vi "Validate Incoming Packet.vi"(8 "error in (no error)":errorcluster, 10 "ControlPacket":refnum<class "ControlPacket.lvclass">, 11 "Session.Server in":refnum<class "Session.Server.lvclass">) -> (0 "error out":errorcluster, 2 "ControlPacket out":refnum<class "ControlPacket.lvclass">, 3 "Session.Server out":refnum<class "Session.Server.lvclass">)   [LabVIEW 2013, in "MQTT Server.lvlib" / "Session.Server.lvclass"]
uses:
  Session.Server.lvclass
  <vilib>/LabVIEW Open Source Project/MQTT Control Packets/Control Packets/ControlPacket/ControlPacket.lvclass
  Session.Server.lvclass/Session.Server.ctl
  <vilib>/LabVIEW Open Source Project/MQTT Control Packets/Control Packets/CONNECT/CONNECT.lvclass
  MQTT_Base/Session/Session.lvclass/Session.ctl
  MQTT_Base/Session/Session.lvclass
  <vilib>/LabVIEW Open Source Project/MQTT Control Packets/Control Packets/SUBSCRIBE/SUBSCRIBE.lvclass
  StoredSessions/StoredSessions.lvclass
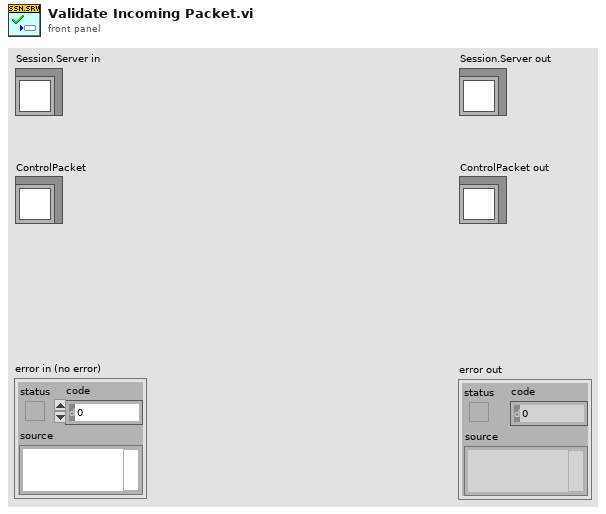
[diagram p1: front panel]
types:
  T1 = typedef "MQTT_Control_Packets.lvlib/ControlPacket.lvclass/Control Packet Type -- enum.ctl" = enum16{"Reserved", "CONNECT", "CONNACK", "PUBLISH", "PUBACK", "PUBREC", "PUBREL", "PUBCOMP", "SUBSCRIBE", "SUBACK", "UNSUBSCRIBE", "UNSUBACK", "PINGREQ", "PINGRESP", "DISCONNECT", "AUTH"}
  T2 = typedef "MQTT_Control_Packets.lvlib/CONNECT.lvclass/ConnectFlags -- cluster.ctl" = cluster{"Reserved":bool, "Clean Session":bool, "Will Flag":bool, "Will QoS 1":bool, "Will QoS 2":bool, "Will Retain":bool, "Password Flag":bool, "User Name Flag":bool}
  T3 = typedef "MQTT_Control_Packets.lvlib/SUBSCRIBE.lvclass/Topic Subscription -- cluster.ctl" = cluster{"Topic Filter":string, "QoS":T4}
  T4 = typedef "MQTT_Control_Packets.lvlib/ControlPacket.lvclass/QualityOfService -- enum.ctl" = enum16{"0 (At Most Once)", "1 (At Least Once)", "2 (Exactly Once)"}
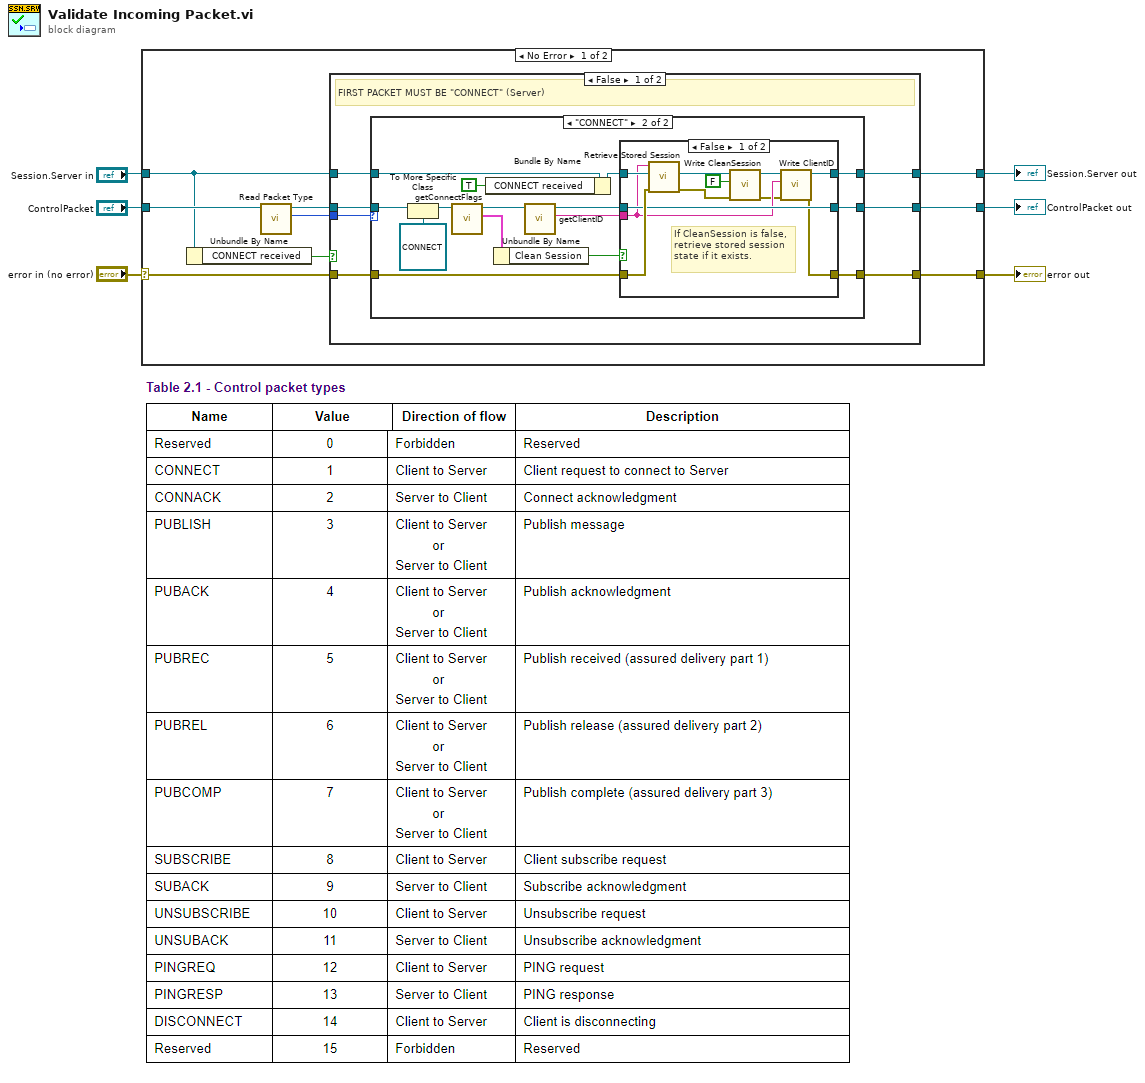
[diagram p0: block diagram]
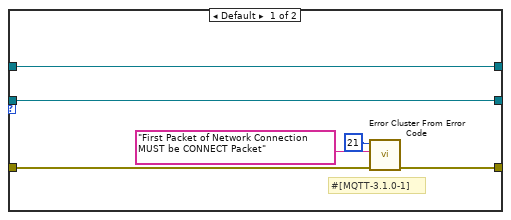
[diagram p2: hidden frame]
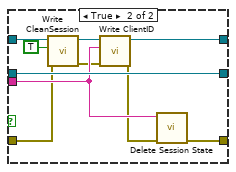
[diagram p3: hidden frame]
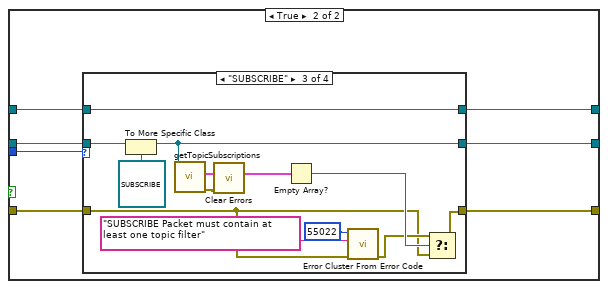
[diagram p4: hidden frame]
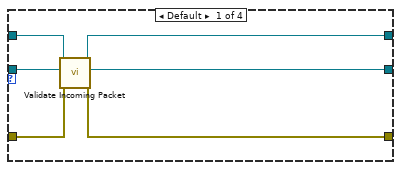
[diagram p5: hidden frame]
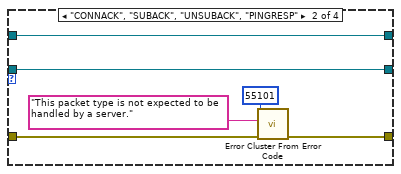
[diagram p6: hidden frame]
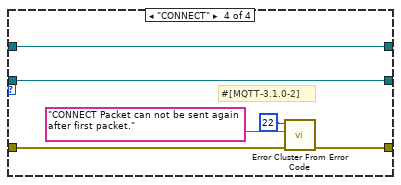
[diagram p7: hidden frame]
diagram:
  n1 = case shown="No Error" "error in (no error)" {
    selector: "error in (no error)" -> [w12 w104]
    tunnel: [w11 w104] -> w1
    tunnel: [w13 w103] -> w3
    tunnel: "Session.Server in" -> [w10 w103]
    tunnel: "ControlPacket" -> [w14 w102]
    tunnel: [w15 w102] -> w2
    frame No Error {
      n2 = Unbundle By Name(w10) -> ("CONNECT received"=w9:bool)
      n3 = call <vilib>:"Read Packet Type.vi"("ControlPacket in"=w14) -> ("Control Packet Type"=w7:T1, "ControlPacket out"=w8:refnum<class "ControlPacket.lvclass">)  [unwired: 9 in]
      n4 = case shown="False" w9 {
        tunnel: w8 -> [w16 w70]
        tunnel: [w17 w69] -> w15
        tunnel: w10 -> [w19 w66]
        tunnel: w7 -> [w20 w71]
        tunnel: [w18 w65] -> w13
        tunnel: w12 -> [w22 w68]
        tunnel: [w21 w67] -> w11
        frame False {
          # "FIRST PACKET MUST BE \"CONNECT\" (Server)"
          n5 = case shown="\"CONNECT\"" w20 {
            tunnel: w22 -> [w27 w32]
            tunnel: [w28 w33] -> w21
            tunnel: w19 -> [w26 w43]
            tunnel: [w26 w36] -> w18
            tunnel: [w25 w34] -> w17
            tunnel: w16 -> [w25 w40]
            frame Default {
              # "#[MQTT-3.1.0-1]"
              n6 = call <vilib>:"Error Cluster From Error Code.vi"("error in (no error)"=w27, "error message (\"\")"="First Packet of Network Connection MUST be CONNECT Packet", "error code (0)"=21) -> ("error out"=w28:errorcluster)  [unwired: 6 in]
            }
            frame "CONNECT" {
              n7 = To More Specific Class(target class=refnum<class "CONNECT.lvclass"> refnum ("CONNECT.lvclass"), reference=w40) -> (specific class reference=w39:refnum<class "CONNECT.lvclass">)  [unwired: 1 in, 1 out]
              n8 = call <vilib>:"getConnectFlags.vi"("CONNECT in"=w39) -> ("Connect Flags"=w38:T2, "CONNECT out"=w31:refnum<class "CONNECT.lvclass">)  [unwired: 9 in]
              n9 = Bundle By Name(cluster=w43, "CONNECT received"=TRUE) -> (w35:refnum<class "Session.Server.lvclass">)
              n10 = Unbundle By Name(w38) -> ("Clean Session"=w37:bool)
              n11 = call <vilib>:"getClientID.vi"("CONNECT in"=w31) -> ("Client ID"=w29:string, "CONNECT out"=w30:refnum<class "CONNECT.lvclass">)  [unwired: 9 in]
              n12 = case shown="False" w37 {
                tunnel: w30 -> [w50 w64]
                tunnel: [w47 w58] -> w36
                tunnel: w35 -> [w54 w62]
                tunnel: [w50 w64] -> w34
                tunnel: [w44 w63] -> w33
                tunnel: w32 -> [w52 w56]
                tunnel: w29 -> [w46 w60]
                frame False {
                  # "If CleanSession is false,\nretrieve stored session\nstate if it exists."
                  n13 = call "Retrieve Stored Session.vi"("error in (no error)"=w52, "Session in"=w54, "Client ID"=w46) -> ("error out"=w51:errorcluster, "Retrieved Session"=w53:refnum<class "Session.Server.lvclass">)  [unwired: 6 in, 1 out]
                  n14 = call "Write CleanSession.vi"("error in (no error)"=w51, "CleanSession"=FALSE, "Session in"=w53) -> ("error out"=w45:errorcluster, "Session out"=w48:refnum<class "Session.Server.lvclass">)  [unwired: 7 in]
                  n15 = call "Write ClientID.vi"("error in (no error)"=w45, "Client ID"=w46, "Session in"=w48) -> ("error out"=w44:errorcluster, "Session out"=w47:refnum<class "Session.Server.lvclass">)  [unwired: 7 in]
                }
                frame True {
                  n16 = call "Write CleanSession.vi"("error in (no error)"=w56, "CleanSession"=TRUE, "Session in"=w62) -> ("error out"=w57:errorcluster, "Session out"=w59:refnum<class "Session.Server.lvclass">)  [unwired: 7 in]
                  n17 = call "Write ClientID.vi"("error in (no error)"=w57, "Client ID"=w60, "Session in"=w59) -> ("error out"=w55:errorcluster, "Session out"=w58:refnum<class "Session.Server.lvclass">)  [unwired: 7 in]
                  n18 = call "Delete Session State.vi"("error in (no error)"=w55, "Client ID"=w60) -> ("error out"=w63:errorcluster)  [unwired: 9 in]
                }
              }
            }
          }
        }
        frame True {
          n19 = case shown="\"SUBSCRIBE\"" w71 {
            tunnel: w70 -> [w77 w82 w95 w99]
            tunnel: [w76 w82 w93 w99] -> w69
            tunnel: w68 -> [w74 w79 w87 w98]
            tunnel: [w73 w80 w84 w97] -> w67
            tunnel: w66 -> [w75 w83 w85 w96]
            tunnel: [w72 w83 w85 w96] -> w65
            frame Default {
              n20 = call-parent "Validate Incoming Packet.vi"("error in (no error)"=w74, "ControlPacket"=w77, "Session in"=w75) -> ("error out"=w73:errorcluster, "ControlPacket out"=w76:refnum<class "ControlPacket.lvclass">, "Session out"=w72:refnum<class "Session.Server.lvclass">)  [unwired: 6 in]
            }
            frame "CONNACK", "SUBACK", "UNSUBACK", "PINGRESP" {
              n21 = call <vilib>:"Error Cluster From Error Code.vi"("error in (no error)"=w79, "error message (\"\")"="This packet type is not expected to be handled by a server.", "error code (0)"=55101) -> ("error out"=w80:errorcluster)  [unwired: 6 in]
            }
            frame "SUBSCRIBE" {
              n22 = To More Specific Class(target class=refnum<class "SUBSCRIBE.lvclass"> refnum ("SUBSCRIBE.lvclass"), reference=w95) -> (specific class reference=w93:refnum<class "SUBSCRIBE.lvclass">)  [unwired: 1 in, 1 out]
              n23 = call <vilib>:"getTopicSubscriptions.vi"("SUBSCRIBE in"=w93) -> ("error out"=w86:errorcluster, "Topic Subscriptions"=w92:T3[])  [unwired: 8 in, 1 out]
              n24 = call <vilib>:"Clear Errors.vi"("error in (no error)"=w86) -> ()  [unwired: 6 in, 1 out]
              n25 = Empty Array?(array=w92) -> (empty?=w89:bool)
              n26 = call <vilib>:"Error Cluster From Error Code.vi"("error in (no error)"=w87, "error message (\"\")"="SUBSCRIBE Packet must contain at least one topic filter", "error code (0)"=55022) -> ("error out"=w88:errorcluster)  [unwired: 6 in]
              n27 = Select(t=w88, s=w89, f=w87) -> (s? t:f=w84:errorcluster)
            }
            frame "CONNECT" {
              # "#[MQTT-3.1.0-2]"
              n28 = call <vilib>:"Error Cluster From Error Code.vi"("error in (no error)"=w98, "error message (\"\")"="CONNECT Packet can not be sent again after first packet.", "error code (0)"=22) -> ("error out"=w97:errorcluster)  [unwired: 6 in]
            }
          }
        }
      }
    }
    frame Error {
    }
  }
  "error out" <- w1
  "Session.Server out" <- w3
  "ControlPacket out" <- w2
